vi "17-xVelToPos.vi"(1 "x velocity":dbl) -> (0 "x position":dbl)   [LabVIEW 2019, in "17.lvlib"]
uses:
  17.lvlib
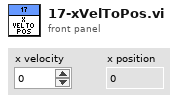
[diagram p1: front panel]
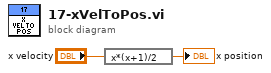
[diagram p0: block diagram]
diagram:
  n1 = expression code="x*(x+1)/2"("x velocity") -> (→"x position":dbl)
